vi "sub_SDR_mimo_DemuxPorts.vi"(4 "Mux in":cdb[][](array[numeric])) -> (0 "Port 2 out":cdb[](array[numeric]), 2 "Port 1 out":cdb[](array[numeric]))   [LabVIEW 2012]
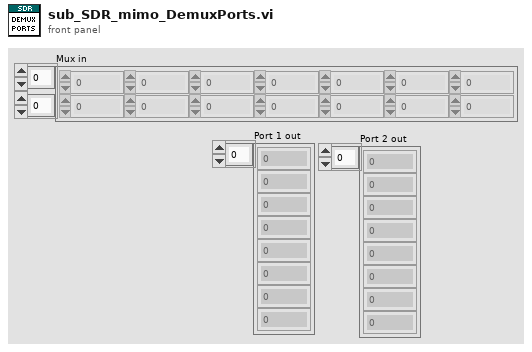
[diagram p1: front panel]
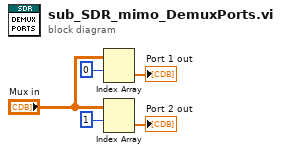
[diagram p0: block diagram]
diagram:
  n1 = Index Array(array="Mux in", index (row)=0 ("index")) -> (element=→"Port 1 out":cdb[])  [unwired: 1 in]
  n2 = Index Array(array="Mux in", index (row)=1 ("index")) -> (element=→"Port 2 out":cdb[])  [unwired: 1 in]
